vi "Instrument List.vi"(10 "All":bool, 11 "Instrument Control Switches":T1) -> (3 "Instrument Names":string[](array[string]))   [LabVIEW 2014, in "Instrument Launcher.lvlib"]
uses:
  controls/Instrument Control Switches.ctl
  Instrument Launcher.lvlib
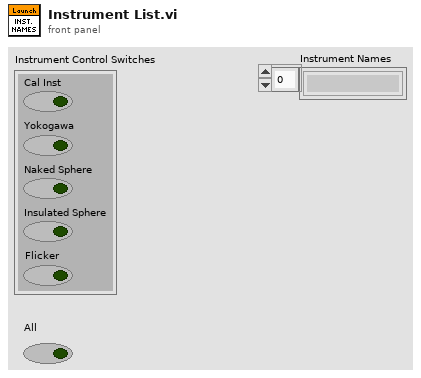
[diagram p1: front panel]
types:
  T1 = typedef "Instrument Control Switches.ctl" = cluster{"Cal Inst":bool, "Yokogawa":bool, "Naked Sphere":bool, "Insulated Sphere":bool, "Flicker":bool}
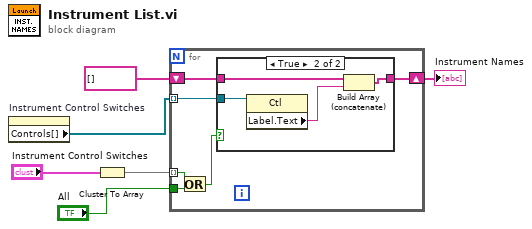
[diagram p0: block diagram]
diagram:
  n1 = property on="Instrument Control Switches" class="Clust (strict)"() -> ("Controls[]"=w2:refnum<vi>[])  [unwired: 2 in, 2 out]
  n2 = Cluster To Array(cluster="Instrument Control Switches") -> (array=w4:bool[])
  n3 = for {
    shift-right: [w12] -> w5
    shift-left: string[] [] -> [w11]
    tunnel: w4 -> [w9] mode=indexing
    tunnel: w2 -> [w10] mode=indexing
    tunnel: "All" -> [w8]
    n4 = Or(x=w9, y=w8) -> (x .or. y?=w7:bool)
    n5 = case shown="True" w7 {
      tunnel: [w13 w17] -> w12
      tunnel: w11 -> [w13 w15]
      tunnel: w10 -> [_ w14]
      frame False {
      }
      frame True {
        n6 = property class="Ctl"(reference=w14) -> ("Label.Text"=w16:string)  [unwired: 1 in, 2 out]
        n7 = Build Array (concatenate)(w15, w16) -> (w17:string[])
      }
    }
  }
  "Instrument Names" <- w5
